vi "Init Refs.vi"(10 "Refs":T1) -> (2 "Refs":refnum<class "Refs.lvclass">)   [LabVIEW 2020, in "_Template.lvlib" / "Templates.lvlib" / "TEMPLATE jettl Actor.lvlib" / "TEMPLATE Actor.lvlib" / "TEMPLATE Refs.lvlib"]
uses:
  TEMPLATE Refs.lvlib
  jettl/jettl/Refs/Refs.lvclass
  TEMPLATE Refs/TEMPLATE Refs.lvclass
  Refs.ctl
panel:
  # "This front panel should not be manipulated."
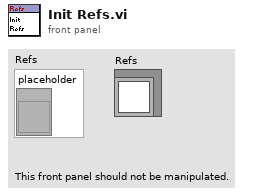
[diagram p1: front panel]
types:
  T1 = typedef "_Template.lvlib/Templates.lvlib/TEMPLATE jettl Actor.lvlib/TEMPLATE Actor.lvlib/TEMPLATE Refs.lvlib/Refs.ctl" = cluster{"placeholder":refnum<vi>}
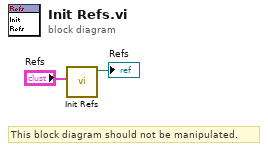
[diagram p0: block diagram]
diagram:
  # "This block diagram should not be manipulated."
  n1 = call "Init Refs.vi"("Refs"="Refs") -> ("TEMPLATE Refs out"=→"Refs":refnum<class "TEMPLATE Refs.lvclass">)  [unwired: 10 in]
